vi "ReadSpreadsheet.vi"() -> ()   [LabVIEW 2017]
uses:
  <vilib>/Utility/file.llb/Read Delimited Spreadsheet (string).vi
  <vilib>/Utility/file.llb/Read Delimited Spreadsheet (DBL).vi
panel:
  in  "Take Screenshot! 2":bool
  in  "Screenshot prefix 2":string="Graph1"
  in  "log/linear  2":bool=TRUE
  out "all data 2":dbl[][](array[numeric]) format="%#_14g"
  in  "file path (dialog if empty) 2":path=path "C:/LabVIEW/DATA/Precooling/MeasureBuildup_20200908_182334_USB6218_RAW.csv"
  out "Graph 2":T1(graph) caption="XY Graph"
  in  "plot every .. measurements":i32=10
  in  "Take Screenshot! 1":bool
  in  "Screenshot prefix 1":string="Graph1"
  in  "Screenshot Base Path":path=path "C:/LabVIEW/DATA/TestData/TestSeries"
  out "Time of Last Measurement":timestamp=timestamp(3679441672.677524 s since 1904-01-01)
  out "error out":errorcluster
  in  "log/linear":bool=TRUE
  out "Graph 1":T1(graph) caption="XY Graph"
  in  "end time":timestamp=timestamp(3682460492.572952 s since 1904-01-01)
  in  "start time":timestamp=timestamp(3682374084.98514 s since 1904-01-01)
  in  "plot":bool
  out "all data 1":dbl[][](array[numeric]) format="%#_14g"
  in  "end":bool
  in  "file path (dialog if empty) 1":path=path "C:/LabVIEW/DATA/Precooling/MeasureBuildup_20200908_182334_USB6218_RAW.csv"
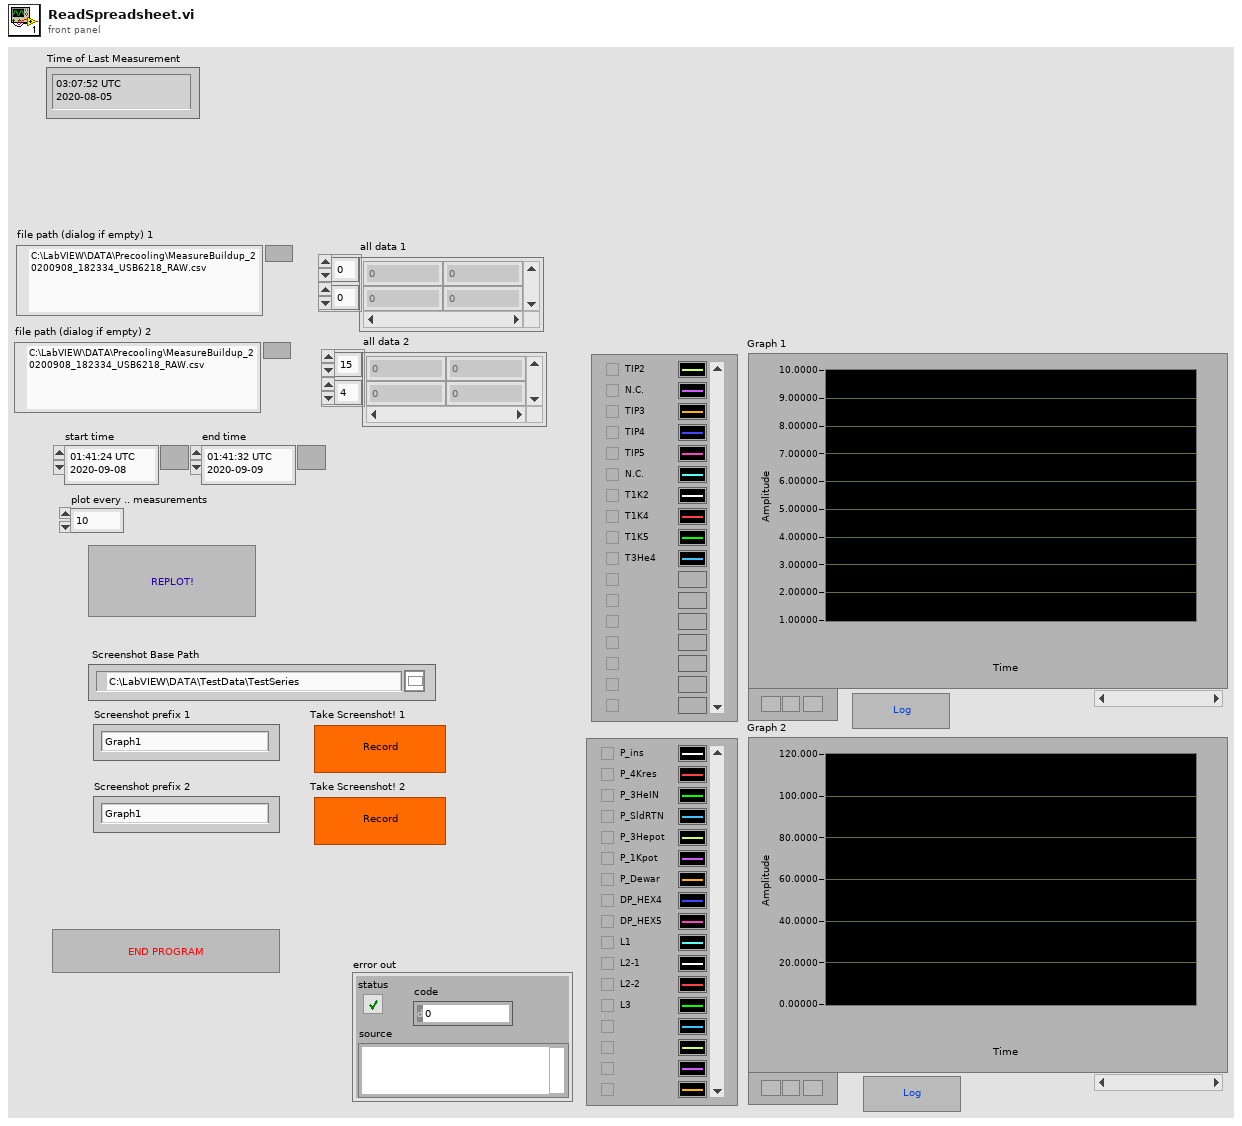
[diagram p1: front panel]
types:
  T1 = cluster{"TimeArray":timestamp[], "DataArrayConv":dbl[]}[]
  T2 = typedef "imagedata.ctl" = cluster{"image type":i32, "image depth":i32, "image":u8[], "mask":u8[], "colors":u32[], "Rectangle":cluster{"left":i16, "top":i16, "right":i16, "bottom":i16}}
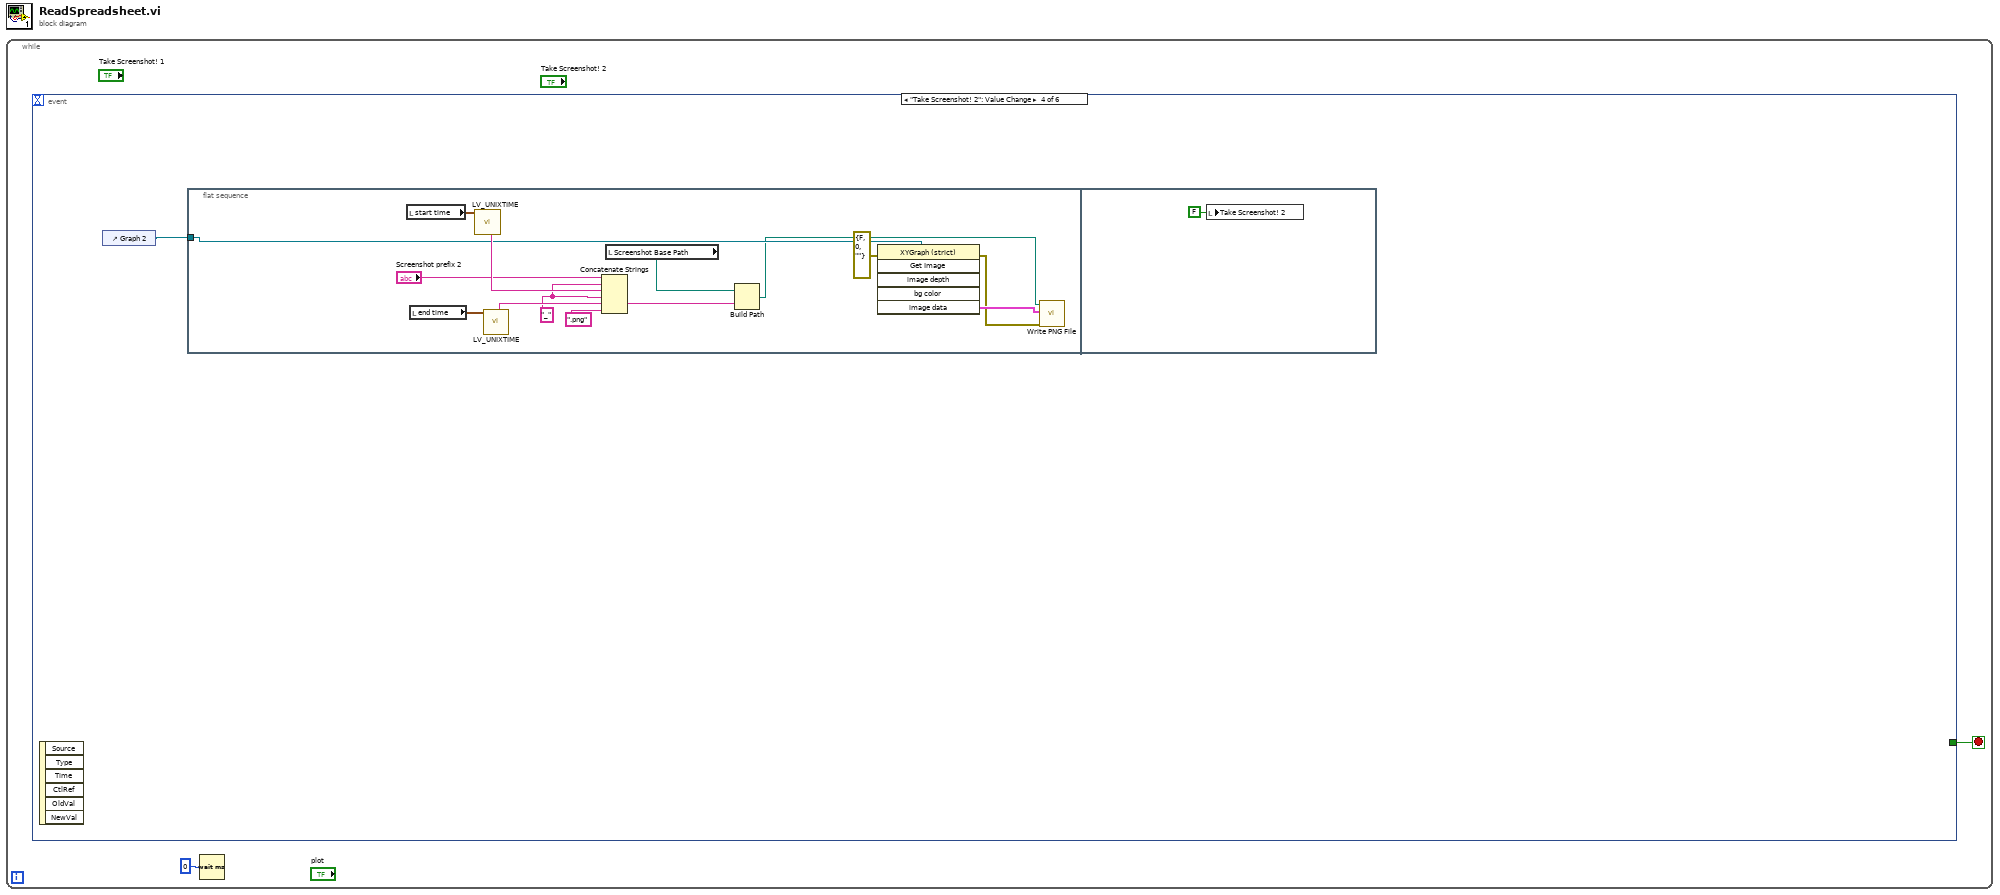
[diagram p0: block diagram]
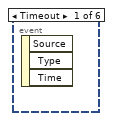
[diagram p2: hidden frame]
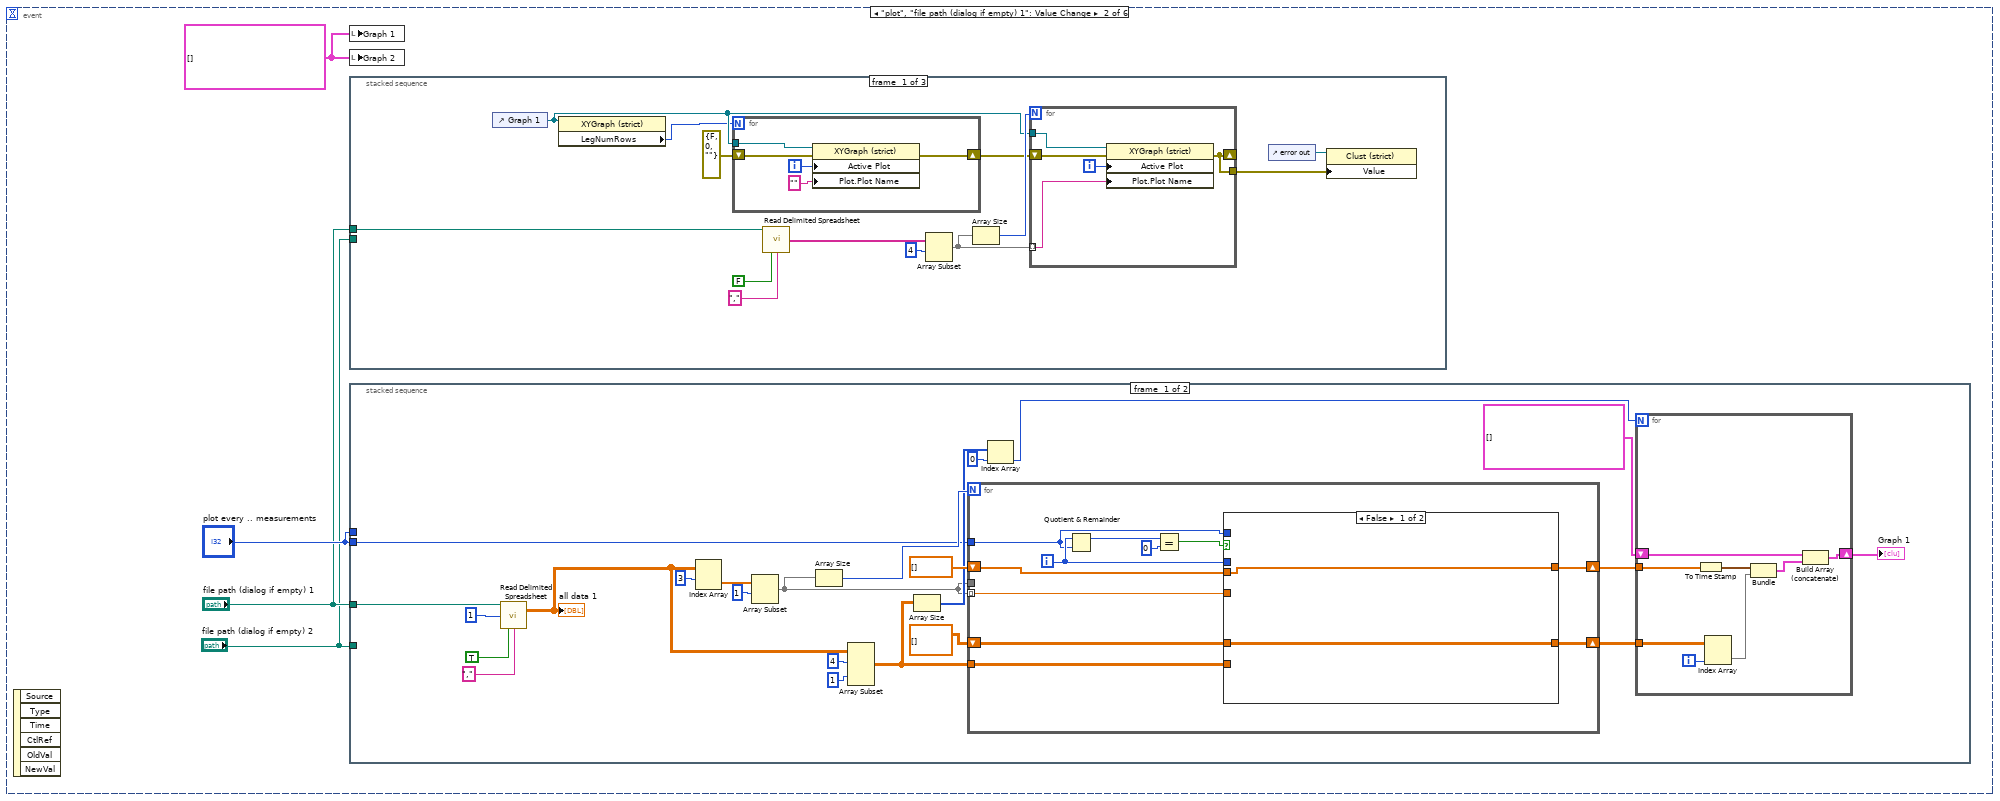
[diagram p3: hidden frame]
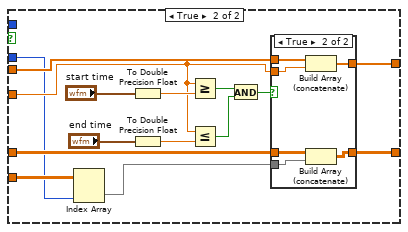
[diagram p4: hidden frame]
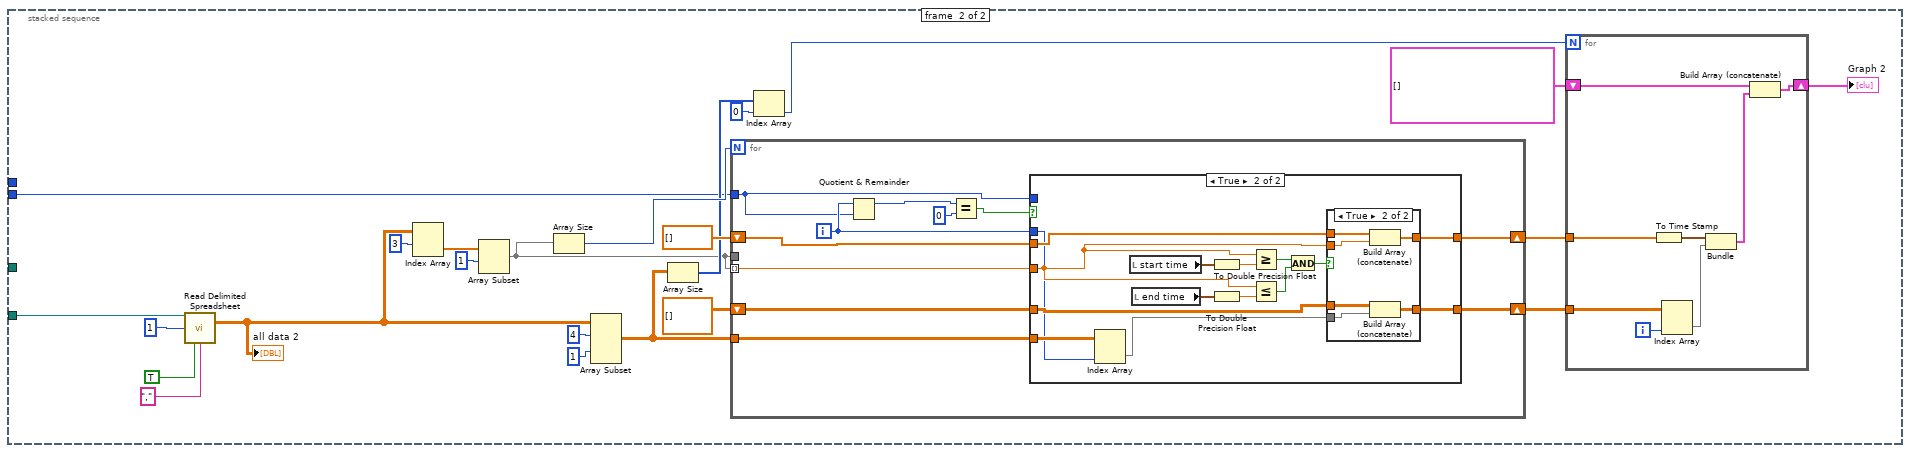
[diagram p6: hidden frame]
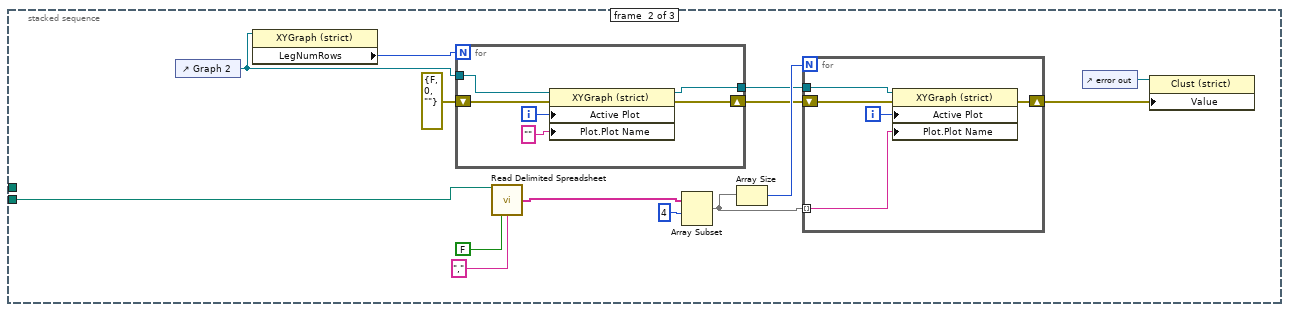
[diagram p9: hidden frame]
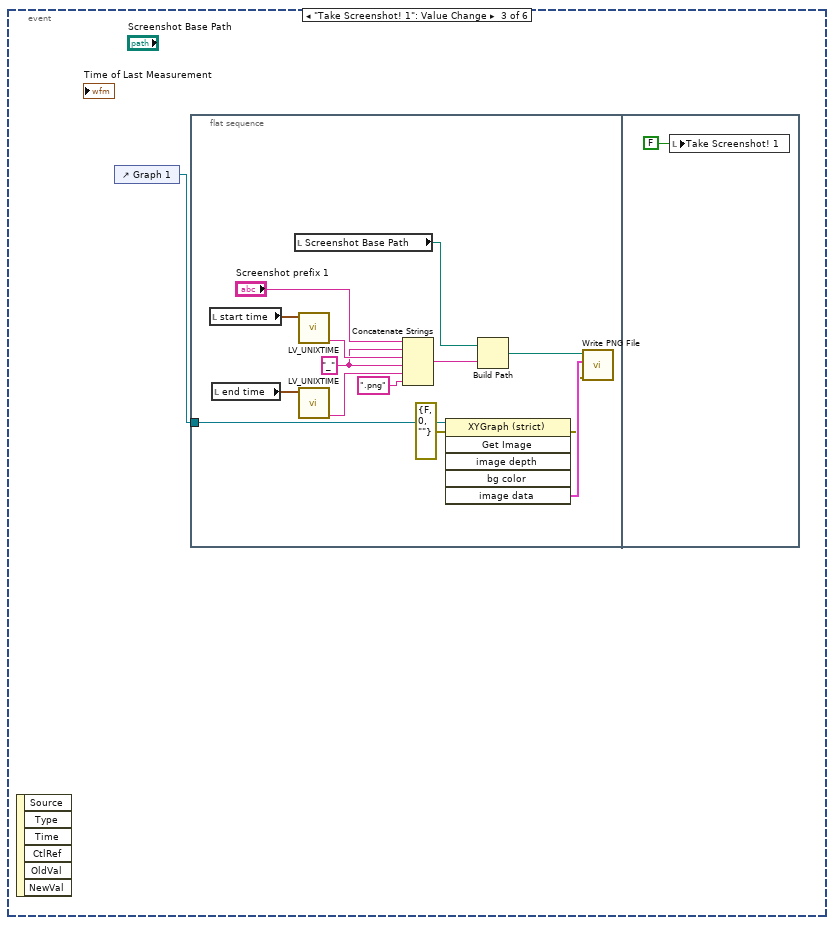
[diagram p11: hidden frame]
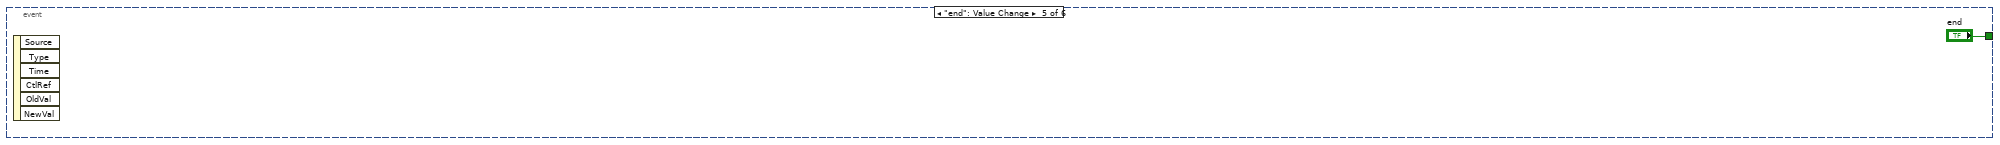
[diagram p12: hidden frame]
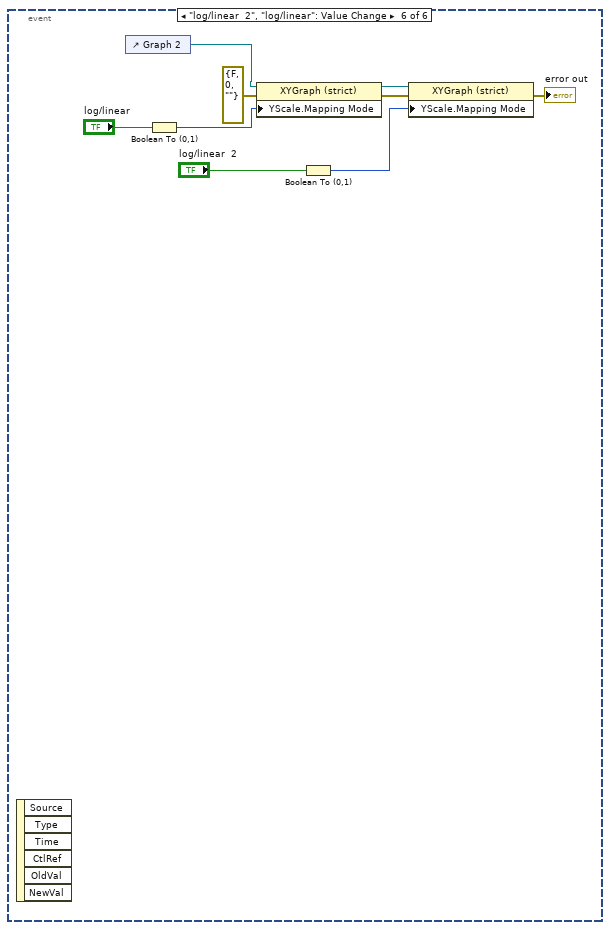
[diagram p13: hidden frame]
diagram:
  n1 = while {
    stop <- w1 stop-if-true
    n2 = event shown="[3] \"Take Screenshot! 2\": Value Change" {
      selector: _ -> [_ _ _ _ _ _]
      dyn-events: _ -> [_ _ _ _ _ _]
      timeout: _ -> [_ _ _ _ _ _]
      tunnel: [_ _ _ _ "end" _] -> w1
      event Timeout {
        n3 = event-data() -> ()  [unwired: 1 in, 3 out]
      }
      event "plot", "file path (dialog if empty) 1": Value Change {
        w6 = T1 [] ("appended array")
        n4 = event-data() -> ()  [unwired: 1 in, 6 out]
        n5 = local write "Graph 1"(w6) -> ()
        n6 = local write "Graph 2"(w6) -> ()
        n7 = stacked-sequence {
          tunnel: "file path (dialog if empty) 1" -> [w144 _ _]
          tunnel: "file path (dialog if empty) 2" -> [_ w167 _]
          frame #0 {
            n8 = control-ref of="Graph 1"() -> (w148:refnum<vi>)
            n9 = property class="XYGraph (strict)"(reference=w148) -> ("LegNumRows"=w147:u32)  [unwired: 1 in, 2 out]
            n10 = for {
              N: w147 -> [_]
              shift-right: [w160] -> w151
              shift-left: errorcluster {"status"=FALSE, "code"=0, "source"=""} ("error in (no error)") -> [w161]
              tunnel: w148 -> [w159]
              i -> [w163]
              n11 = property class="XYGraph (strict)"(reference=w159, error in=w161, "Active Plot"=w163, "Plot.Plot Name"="") -> (error out=w160:errorcluster)  [unwired: 1 out]
            }
            n12 = call-poly <vilib>:"Read Delimited Spreadsheet.vi"("file path (dialog if empty)"=w144, "transpose? (F)"=FALSE, "delimiter (\\t)"="," ("delimiter (\\t)")) -> ("first row"=w146:string[])  [unwired: 7 in, 5 out]
            n13 = Array Subset(array=w146, index=4) -> (w142:string[])  [unwired: 1 in]
            n14 = Array Size(array=w142) -> (size(s)=w153:i32)
            n15 = for {
              N: w153 -> [_]
              shift-right: [w156] -> _
              shift-left: w151 -> [w157]
              tunnel: [w156] -> w150
              tunnel: w142 -> [w155] mode=indexing
              tunnel: w148 -> [w154]
              i -> [w158]
              n16 = property class="XYGraph (strict)"(reference=w154, error in=w157, "Active Plot"=w158, "Plot.Plot Name"=w155) -> (error out=w156:errorcluster)  [unwired: 1 out]
            }
            n17 = control-ref of="error out"() -> (w149:refnum<vi>)
            n18 = property class="Clust (strict)"(reference=w149, "Value"=w150) -> ()  [unwired: 1 in, 2 out]
          }
          frame #1 {
            n19 = control-ref of="Graph 2"() -> (w171:refnum<vi>)
            n20 = property class="XYGraph (strict)"(reference=w171) -> ("LegNumRows"=w170:u32)  [unwired: 1 in, 2 out]
            n21 = for {
              N: w170 -> [_]
              shift-right: [w185] -> w175
              shift-left: errorcluster {"status"=FALSE, "code"=0, "source"=""} ("error in (no error)") -> [w186]
              tunnel: w171 -> [w184]
              tunnel: [w183] -> w172
              i -> [w188]
              n22 = property class="XYGraph (strict)"(reference=w184, error in=w186, "Active Plot"=w188, "Plot.Plot Name"="") -> (reference out=w183:refnum<vi>, error out=w185:errorcluster)
            }
            n23 = call-poly <vilib>:"Read Delimited Spreadsheet.vi"("file path (dialog if empty)"=w167, "transpose? (F)"=FALSE, "delimiter (\\t)"="," ("delimiter (\\t)")) -> ("first row"=w165:string[])  [unwired: 7 in, 5 out]
            n24 = Array Subset(array=w165, index=4) -> (w164:string[])  [unwired: 1 in]
            n25 = Array Size(array=w164) -> (size(s)=w177:i32)
            n26 = for {
              N: w177 -> [_]
              shift-right: [w180] -> w173
              shift-left: w175 -> [w181]
              tunnel: w172 -> [w179]
              tunnel: w164 -> [w178] mode=indexing
              i -> [w182]
              n27 = property class="XYGraph (strict)"(reference=w179, error in=w181, "Active Plot"=w182, "Plot.Plot Name"=w178) -> (error out=w180:errorcluster)  [unwired: 1 out]
            }
            n28 = control-ref of="error out"() -> (w174:refnum<vi>)
            n29 = property class="Clust (strict)"(reference=w174, "Value"=w173) -> ()  [unwired: 1 in, 2 out]
          }
          frame #2 {
          }
        }
        n30 = stacked-sequence {
          tunnel: "plot every .. measurements" -> [w8 w76]
          tunnel: "plot every .. measurements" -> [_ _]
          tunnel: "file path (dialog if empty) 2" -> [_ w74]
          tunnel: "file path (dialog if empty) 1" -> [w7 _]
          frame #0 {
            n31 = call-poly <vilib>:"Read Delimited Spreadsheet.vi"("file path (dialog if empty)"=w7, "start of read offset (chars.:0)"=1, "transpose? (F)"=TRUE, "delimiter (\\t)"="," ("delimiter (\\t)")) -> ("all rows"=w21:dbl[][])  [unwired: 6 in, 5 out]
            "all data 1" <- w21
            n32 = Index Array(array=w21, index (row)=3) -> (element=w25:dbl[])  [unwired: 1 in]
            n33 = Array Subset(array=w25, index=1) -> (w10:dbl[])  [unwired: 1 in]
            n34 = Array Size(array=w10) -> (size(s)=w23:i32)
            n35 = Array Subset(array=w21, index (row)=4 ("index"), index (col)=1 ("index")) -> (w18:dbl[][])  [unwired: 2 in]
            n36 = Array Size(array=w18) -> (size(s)=w11:i32[])
            n37 = for {
              N: w23 -> [_]
              tunnel: w10 -> [w39] mode=indexing
              shift-right: [w38] -> w14
              shift-left: dbl[] [] ("datetime array 2") -> [w40]
              shift-right: [w37] -> w13
              shift-left: dbl[][] [] -> [w36]
              tunnel: w18 -> [w35]
              tunnel: w10 -> [_]
              tunnel: w8 -> [w30]
              i -> [w34]
              n38 = Quotient & Remainder(x=w34, y=w30) -> (x-y*floor(x/y)=w33:i32)  [unwired: 1 out]
              n39 = Equal?(x=w33, y=0) -> (x = y?=w31:bool)
              n40 = case shown="False" w31 {
                tunnel: w40 -> [w42 w50]
                tunnel: w39 -> [_ w49]
                tunnel: [w42 w48] -> w38
                tunnel: [w41 w47] -> w37
                tunnel: w36 -> [w41 w46]
                tunnel: w35 -> [_ w45]
                tunnel: w34 -> [_ w43]
                tunnel: w30 -> [_ _]
                frame False {
                }
                frame True {
                  n41 = Index Array(array=w45, index (col)=w43) -> (element=w44:dbl[])  [unwired: 1 in]
                  n42 = To Double Precision Float(number="start time") -> (double precision float=w56:dbl)
                  n43 = To Double Precision Float(number="end time") -> (double precision float=w55:dbl)
                  n44 = Greater Or Equal?(x=w49, y=w56) -> (x >= y?=w53:bool)
                  n45 = Less Or Equal?(x=w49, y=w55) -> (x <= y?=w52:bool)
                  n46 = And(x=w53, y=w52) -> (x .and. y?=w51:bool)
                  n47 = case shown="True" w51 {
                    tunnel: [w59 w65] -> w48
                    tunnel: w50 -> [w59 w63]
                    tunnel: w49 -> [_ w64]
                    tunnel: w44 -> [_ w62]
                    tunnel: [w58 w61] -> w47
                    tunnel: w46 -> [w58 w60]
                    frame False {
                    }
                    frame True {
                      n48 = Build Array (concatenate)(w63, w64) -> (w65:dbl[])
                      n49 = Build Array (concatenate)(w60, w62) -> (w61:dbl[][])
                    }
                  }
                }
              }
            }
            n50 = Index Array(array=w11, index=0) -> (element=w15:i32)
            n51 = for {
              N: w15 -> [_]
              tunnel: w14 -> [w71]
              tunnel: w13 -> [w73]
              shift-right: [w68] -> w9
              shift-left: T1 [] ("appended array") -> [w69]
              i -> [w66]
              n52 = To Time Stamp(1:w71) -> (0:w70:timestamp[])
              n53 = Index Array(array=w73, index (col)=w66) -> (element=w72:dbl[])  [unwired: 1 in]
              n54 = Bundle(w70, w72) -> (w67:cluster{timestamp[], dbl[]})  [unwired: 1 in]
              n55 = Build Array (concatenate)(w69, w67) -> (w68:T1)
            }
            "Graph 1" <- w9
          }
          frame #1 {
            n56 = call-poly <vilib>:"Read Delimited Spreadsheet.vi"("file path (dialog if empty)"=w74, "start of read offset (chars.:0)"=1, "transpose? (F)"=TRUE, "delimiter (\\t)"="," ("delimiter (\\t)")) -> ("all rows"=w88:dbl[][])  [unwired: 6 in, 5 out]
            "all data 2" <- w88
            n57 = Index Array(array=w88, index (row)=3) -> (element=w92:dbl[])  [unwired: 1 in]
            n58 = Array Subset(array=w92, index=1) -> (w77:dbl[])  [unwired: 1 in]
            n59 = Array Size(array=w77) -> (size(s)=w90:i32)
            n60 = Array Subset(array=w88, index (row)=4 ("index"), index (col)=1 ("index")) -> (w85:dbl[][])  [unwired: 2 in]
            n61 = Array Size(array=w85) -> (size(s)=w78:i32[])
            n62 = for {
              N: w90 -> [_]
              tunnel: w77 -> [w106] mode=indexing
              shift-right: [w105] -> w81
              shift-left: dbl[] [] ("datetime array 2") -> [w107]
              shift-right: [w104] -> w80
              shift-left: dbl[][] [] -> [w103]
              tunnel: w85 -> [w102]
              tunnel: w77 -> [_]
              tunnel: w76 -> [w97]
              i -> [w101]
              n63 = Quotient & Remainder(x=w101, y=w97) -> (x-y*floor(x/y)=w100:i32)  [unwired: 1 out]
              n64 = Equal?(x=w100, y=0) -> (x = y?=w98:bool)
              n65 = case shown="True" w98 {
                tunnel: w107 -> [w109 w119]
                tunnel: w106 -> [_ w118]
                tunnel: [w109 w117] -> w105
                tunnel: [w108 w116] -> w104
                tunnel: w103 -> [w108 w115]
                tunnel: w102 -> [_ w114]
                tunnel: w101 -> [_ w112]
                tunnel: w97 -> [_ _]
                frame False {
                }
                frame True {
                  n66 = Index Array(array=w114, index (col)=w112) -> (element=w113:dbl[])  [unwired: 1 in]
                  n67 = local read "start time"() -> (w110:timestamp)
                  n68 = local read "end time"() -> (w111:timestamp)
                  n69 = To Double Precision Float(number=w110) -> (double precision float=w124:dbl)
                  n70 = To Double Precision Float(number=w111) -> (double precision float=w123:dbl)
                  n71 = Greater Or Equal?(x=w118, y=w124) -> (x >= y?=w122:bool)
                  n72 = Less Or Equal?(x=w118, y=w123) -> (x <= y?=w121:bool)
                  n73 = And(x=w122, y=w121) -> (x .and. y?=w120:bool)
                  n74 = case shown="True" w120 {
                    tunnel: [w126 w132] -> w117
                    tunnel: w119 -> [w126 w130]
                    tunnel: w118 -> [_ w131]
                    tunnel: w113 -> [_ w129]
                    tunnel: [w125 w128] -> w116
                    tunnel: w115 -> [w125 w127]
                    frame False {
                    }
                    frame True {
                      n75 = Build Array (concatenate)(w130, w131) -> (w132:dbl[])
                      n76 = Build Array (concatenate)(w127, w129) -> (w128:dbl[][])
                    }
                  }
                }
              }
            }
            n77 = Index Array(array=w78, index=0) -> (element=w82:i32)
            n78 = for {
              N: w82 -> [_]
              tunnel: w81 -> [w138]
              tunnel: w80 -> [w140]
              shift-right: [w135] -> w75
              shift-left: T1 [] ("appended array") -> [w136]
              i -> [w133]
              n79 = To Time Stamp(1:w138) -> (0:w137:timestamp[])
              n80 = Index Array(array=w140, index (col)=w133) -> (element=w139:dbl[])  [unwired: 1 in]
              n81 = Bundle(w137, w139) -> (w134:cluster{timestamp[], dbl[]})  [unwired: 1 in]
              n82 = Build Array (concatenate)(w136, w134) -> (w135:T1)
            }
            "Graph 2" <- w75
          }
        }
      }
      event "Take Screenshot! 1": Value Change {
        n83 = event-data() -> ()  [unwired: 1 in, 6 out]
        n84 = control-ref of="Graph 1"() -> (w189:refnum<vi>)
        n85 = flat-sequence {
          tunnel: w189 -> [w194]
          frame #0 {
            w197 = "_" ("string")
            n86 = local read "start time"() -> (w199:timestamp)
            n87 = local read "end time"() -> (w201:timestamp)
            n88 = local read "Screenshot Base Path"() -> (w202:path)
            n89 = call "LV_UNIXTIME.vi"("current time"=w199) -> ("date/time string"=w198:string)  [unwired: 9 in, 1 out]
            n90 = call "LV_UNIXTIME.vi"("current time"=w201) -> ("date/time string"=w200:string)  [unwired: 9 in, 1 out]
            n91 = Concatenate Strings("Screenshot prefix 1", w197, w198, w197, w200, ".png" ("string")) -> (w203:string)
            n92 = invoke class="XYGraph (strict)" method="Get Image"(reference=w194, error in=errorcluster {"status"=FALSE, "code"=0, "source"=""} ("error in (no error)")) -> (error out=w191:errorcluster, "image data"=w192:T2)  [unwired: 4 in, 4 out]
            n93 = Build Path(base path=w202, name or relative path=w203) -> (appended path=w193:path)
            n94 = call <vilib>:"Write PNG File.vi"("error in (no error)"=w191, "image data"=w192, "path to PNG file"=w193) -> ()  [unwired: 7 in, 2 out]
          }
          frame #1 {
            n95 = local write "Take Screenshot! 1"(FALSE ("Take Screenshot! 1")) -> ()
          }
        }
      }
      event "Take Screenshot! 2": Value Change {
        n96 = event-data() -> ()  [unwired: 1 in, 6 out]
        n97 = control-ref of="Graph 2"() -> (w205:refnum<vi>)
        n98 = flat-sequence {
          tunnel: w205 -> [w210]
          frame #0 {
            w212 = "_" ("string")
            n99 = local read "start time"() -> (w215:timestamp)
            n100 = local read "end time"() -> (w217:timestamp)
            n101 = call "LV_UNIXTIME.vi"("current time"=w215) -> ("date/time string"=w214:string)  [unwired: 9 in, 1 out]
            n102 = call "LV_UNIXTIME.vi"("current time"=w217) -> ("date/time string"=w216:string)  [unwired: 9 in, 1 out]
            n103 = Concatenate Strings("Screenshot prefix 2", w212, w214, w212, w216, ".png" ("string")) -> (w219:string)
            n104 = local read "Screenshot Base Path"() -> (w218:path)
            n105 = Build Path(base path=w218, name or relative path=w219) -> (appended path=w208:path)
            n106 = invoke class="XYGraph (strict)" method="Get Image"(reference=w210, error in=errorcluster {"status"=FALSE, "code"=0, "source"=""} ("error in (no error)")) -> (error out=w207:errorcluster, "image data"=w209:T2)  [unwired: 4 in, 4 out]
            n107 = call <vilib>:"Write PNG File.vi"("error in (no error)"=w207, "image data"=w209, "path to PNG file"=w208) -> ()  [unwired: 7 in, 2 out]
          }
          frame #1 {
            n108 = local write "Take Screenshot! 2"(FALSE ("Take Screenshot! 1")) -> ()
          }
        }
      }
      event "end": Value Change {
        n109 = event-data() -> ()  [unwired: 1 in, 6 out]
      }
      event "log/linear  2", "log/linear": Value Change {
        n110 = event-data() -> ()  [unwired: 1 in, 6 out]
        n111 = control-ref of="Graph 2"() -> (w223:refnum<vi>)
        n112 = Boolean To (0,1)(Boolean="log/linear") -> (0, 1=w229:i16)
        n113 = property class="XYGraph (strict)"(reference=w223, error in=errorcluster {"status"=FALSE, "code"=0, "source"=""} ("error in (no error)"), "YScale.Mapping Mode"=w229) -> (reference out=w222:refnum<vi>, error out=w225:errorcluster)
        n114 = Boolean To (0,1)(Boolean="log/linear  2") -> (0, 1=w226:i16)
        n115 = property class="XYGraph (strict)"(reference=w222, error in=w225, "YScale.Mapping Mode"=w226) -> (error out=→"error out":errorcluster)  [unwired: 1 out]
      }
    }
    n116 = Wait (ms)(milliseconds to wait=u32 0) -> ()  [unwired: 1 out]
  }
